vi "flat sequence structure_time to match.vi"() -> ()   [LabVIEW 2016]
panel:
  out "Time to Match":dbl
  out "Number of Iterations":dbl
  out "Current Number":dbl
  in  "Number to Match":dbl
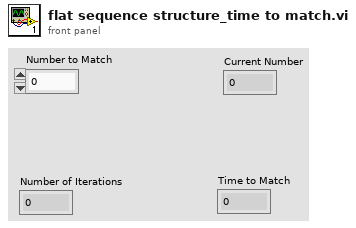
[diagram p1: front panel]
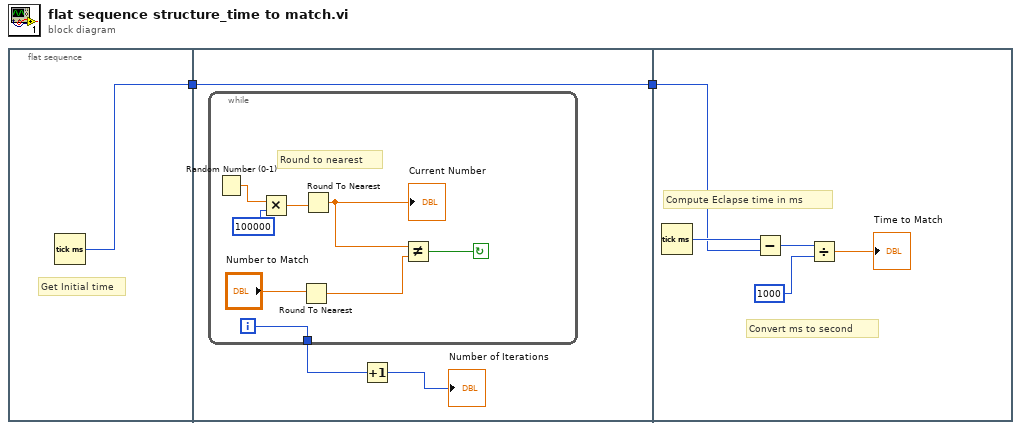
[diagram p0: block diagram]
diagram:
  n1 = flat-sequence {
    tunnel: [w3] -> w1
    tunnel: [w4] -> w2
    tunnel: w1 -> [w4]
    tunnel: w2 -> [w15]
    frame #0 {
      # "Get Initial time"
      n2 = Tick Count (ms)() -> (millisecond timer value=w3:u32)
    }
    frame #1 {
      n3 = while {
        tunnel: [w7] -> w5
        i -> [w7]
        stop <- w8 continue-if-true
        # "Round to nearest"
        n4 = Random Number (0-1)() -> (number: 0 to 1=w14:dbl)
        n5 = Multiply(x=w14, y=100000) -> (x*y=w12:dbl)
        n6 = Round To Nearest(number="Number to Match") -> (nearest integer value=w9:dbl)
        n7 = Round To Nearest(number=w12) -> (nearest integer value=w11:dbl)
        "Current Number" <- w11
        n8 = Not Equal?(x=w11, y=w9) -> (x != y?=w8:bool)
      }
      n9 = Increment(x=w5) -> (x+1=→"Number of Iterations":i32)
    }
    frame #2 {
      # "Convert ms to second"
      # "Compute Eclapse time in ms"
      n10 = Tick Count (ms)() -> (millisecond timer value=w19:u32)
      n11 = Subtract(x=w19, y=w15) -> (x-y=w18:u32)
      n12 = Divide(x=w18, y=1000) -> (x/y=→"Time to Match":dbl)
    }
  }
